vi "mL to steps.vi"(1 "mL in":dbl) -> (0 "steps out":i32)   [LabVIEW 2010]
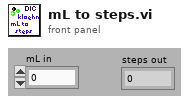
[diagram p1: front panel]
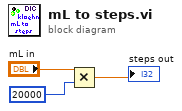
[diagram p0: block diagram]
diagram:
  n1 = Multiply(x="mL in", y=20000) -> (x*y=→"steps out":dbl)
